vi "Count.vi"(0 "Start Count (SR)":i32, 2 "Switch":bool, 11 "Boolean In (SR)":bool) -> (4 "Count (SR)":i32, 15 "Boolean Out (SR)":bool)   [LabVIEW 2017]
doc: "This SubVI counts the number of times the Boolean switch makes a transition from the false state to the true state. To utilize this SubVI in a main VI, the Count Control and Indicator should be connected to an integer shift register (SR) that has been initialized to zero, and the Boolean Control and Indicator should be connected to a Boolean shift register that has been initialized to the false state."
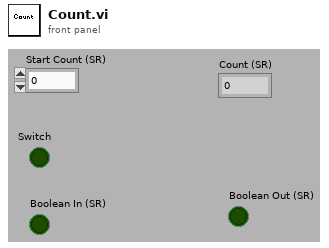
[diagram p1: front panel]
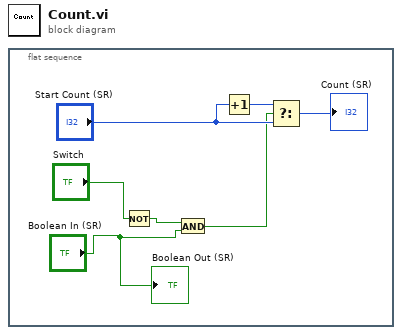
[diagram p0: block diagram]
diagram:
  n1 = flat-sequence {
    frame #0 {
      n2 = Not(x="Switch") -> (.not. x?=w3:bool)
      n3 = And(x=w3, y="Boolean In (SR)") -> (x .and. y?=w1:bool)
      n4 = Increment(x="Start Count (SR)") -> (x+1=w5:i32)
      n5 = Select(t=w5, s=w1, f="Start Count (SR)") -> (s? t:f=→"Count (SR)":i32)
      "Boolean Out (SR)" <- "Boolean In (SR)"
    }
  }
